vi "Parameter XML Write (ni-AIM).vi"(8 "error in":errorcluster, 10 "Parameter Array":T1[](array[typedef]), 11 "parameter file in":refnum<k24>) -> (0 "error out":errorcluster, 3 "parameter file out":refnum<k24>)   [LabVIEW 2020]
uses:
  Controls/Database_Array.ctl
  Controls/Encoding.ctl
  C:/Users/Administrator/Desktop/GIT/Ballard-Arinc-429-XML-Generator/Source/Assemblies/Aim_Parameter_ni/bin/Debug/AIM_429_Parameter_ni.dll
  Assemblies/Aim_Parameter_ni/bin/Debug/AIM_429_Parameter_ni.dll
  Libraries/Aim_Parameter_ni/_tyedefs/label_type.ctl
  Libraries/Aim_Parameter_ni/_tyedefs/parameter_type.ctl
  <userlib>/_OpenG.lib/array/array.llb/Remove Duplicates from 1D Array (I32)__ogtk.vi
  <userlib>/_OpenG.lib/array/array.llb/Filter 1D Array with Scalar (I32)__ogtk.vi
  <userlib>/_OpenG.lib/array/array.llb/Index 1D Array Elements (Variant)__ogtk.vi
  Libraries/Aim_Parameter_ni/AIM_429_Parameter_ni.lvlib
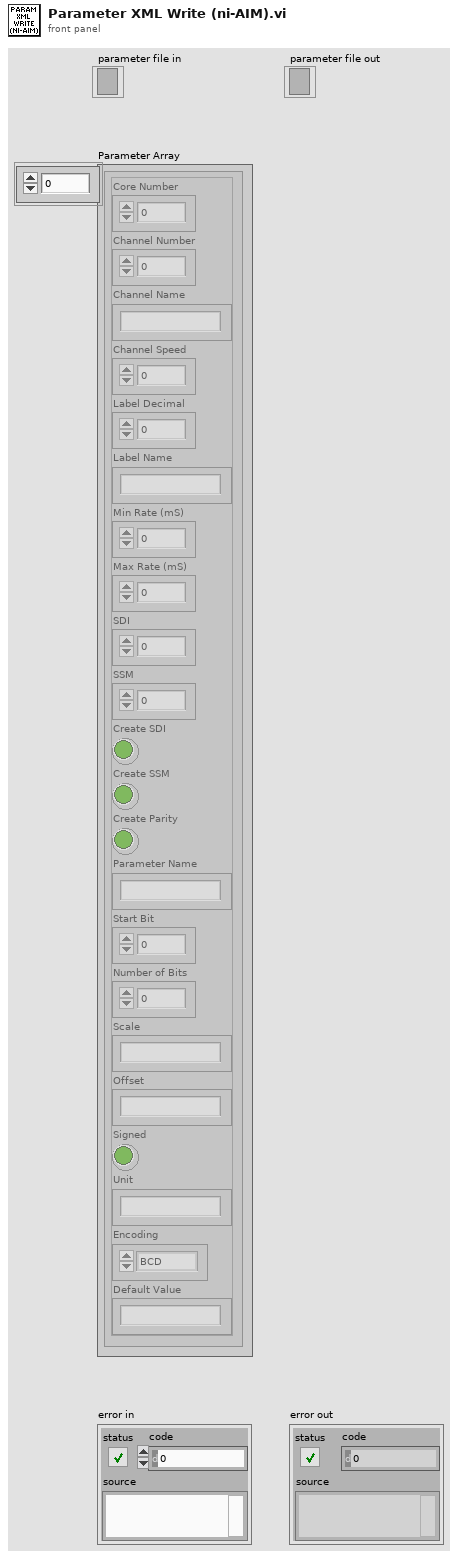
[diagram p1: front panel]
types:
  T1 = typedef "Database_Array.ctl" = cluster{"Core Number":i32, "Channel Number":i32, "Channel Name":string, "Channel Speed":i32, "Label Decimal":i32, "Label Name":string, "Min Rate (mS)":i32, "Max Rate (mS)":i32, "SDI":i32, "SSM":i32, "Create SDI":bool, "Create SSM":bool, "Create Parity":bool, "Parameter Name":string, "Start Bit":i32, "Number of Bits":i32, "Scale":string, "Offset":string, "Signed":bool, "Unit":string, "Encoding":T2, "Default Value":string}
  T2 = typedef "Encoding.ctl" = enum16{"BCD", "BNR", "Discrete"}
  T3 = typedef "AIM_429_Parameter_ni.lvlib/label_type.ctl" = cluster{"createParityChannel":bool, "createSDIChannel":bool, "createSSMChannel":bool, "createTimestampChannel":bool, "labelDecimal":i32, "labelDecimalSpecified":bool, "labelOctal":i32, "labelOctalSpecified":bool, "sdi":i32, "transferType":i32, "period":i32}
  T4 = typedef "AIM_429_Parameter_ni.lvlib/parameter_type.ctl" = cluster{"defaultValue":dbl, "encoding":i32, "name":string, "numberOfBits":i32, "offset":dbl, "scale":dbl, "signed":bool, "startBit":i32, "unit":string}
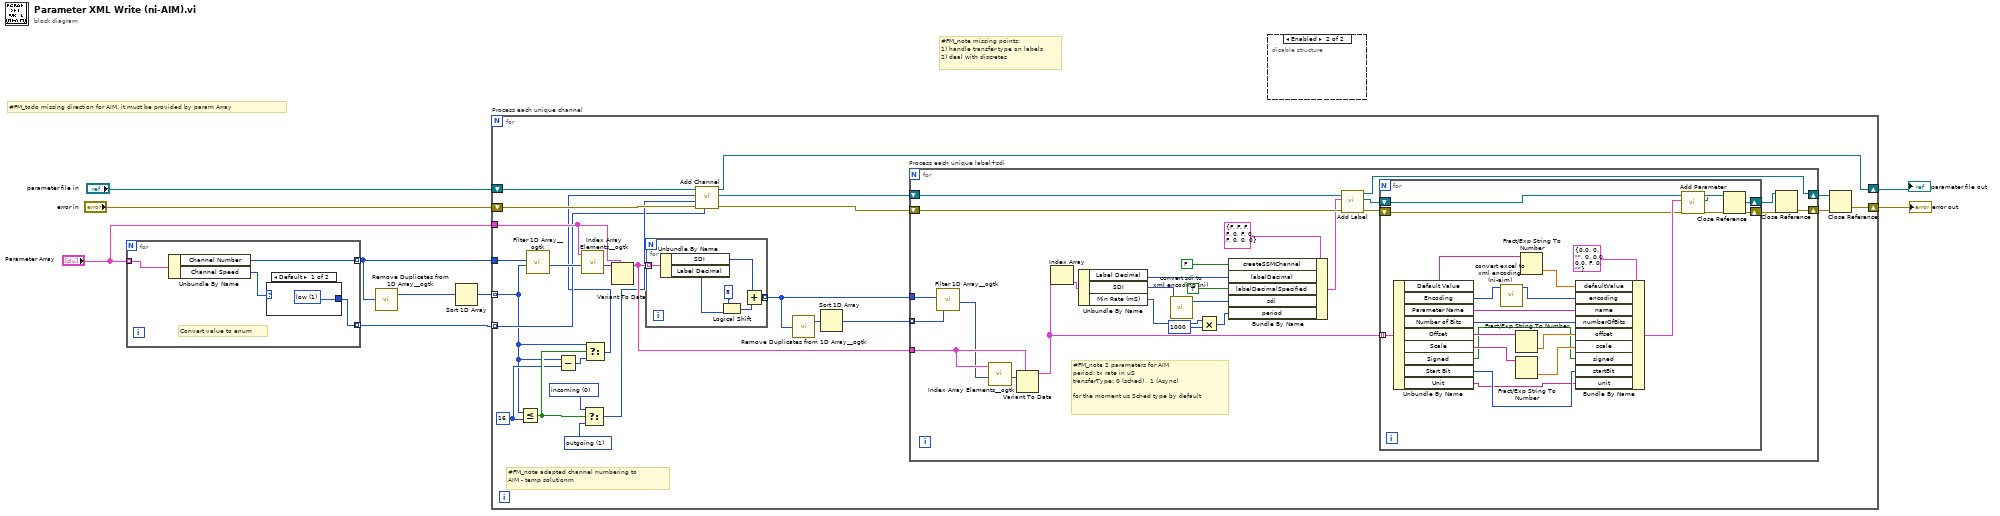
[diagram p0: block diagram]
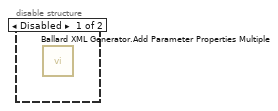
[diagram p2: hidden frame]
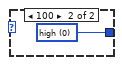
[diagram p3: hidden frame]
diagram:
  # "#FM_todo missing direction for AIM, it must be provided by param Array"
  # "#FM_note missing points:\n1) handle transfer type on labels\n2) deal with discretes"
  n1 = for {
    tunnel: [w13] -> w6 mode=indexing
    tunnel: "Parameter Array" -> [w12] mode=indexing
    tunnel: [w10] -> w1 mode=indexing
    # "Convert value to enum"
    n2 = Unbundle By Name(w12) -> ("Channel Number"=w13:i32, "Channel Speed"=w11:i32)
    n3 = case shown="Default" w11 {
      tunnel: [w14 w15] -> w10
      frame Default {
        w14 = 1 items=["high", "low"] ("speed (high)")
      }
      frame 100 {
        w15 = 0 items=["high", "low"] ("speed (high)")
      }
    }
  }
  n4 = call-poly <userlib>:"Remove Duplicates from 1D Array__ogtk.vi"("Input Array"=w6) -> ("Output Array"=w8:i32[])  [unwired: 1 out]
  n5 = Sort 1D Array(array=w8) -> (sorted array=w9:i32[])
  n6 = for "Process each unique channel" {
    tunnel: w9 -> [w17] mode=indexing
    tunnel: w6 -> [w40]
    tunnel: "Parameter Array" -> [w39]
    shift-right: [w37] -> w3
    shift-left: "parameter file in" -> [w38]
    shift-right: [w35] -> w2
    shift-left: "error in" -> [w36]
    tunnel: w1 -> [w21] mode=indexing
    w24 = 1 items=["incoming", "outgoing"] ("direction")
    w23 = 0 items=["incoming", "outgoing"] ("direction")
    w18 = 16 ("y")
    # "#FM_note adapted channel numbering to \nAIM - temp solutionm"
    n7 = Less Or Equal?(x=w17, y=w18) -> (x <= y?=w20:bool)
    n8 = call-poly <userlib>:"Filter 1D Array__ogtk.vi"("items to filter"=w17, "array"=w40) -> ("filtered item indices"=w31:i32[])  [unwired: 4 in, 1 out]
    n9 = Subtract(x=w17, y=w18) -> (x-y=w19:i32)
    n10 = call-poly <userlib>:"Index Array Elements__ogtk.vi"("indices"=w31, "array"=w39) -> ("elements"=w32:variant[])  [unwired: 9 in]
    n11 = Select(t=w23, s=w20, f=w24) -> (s? t:f=w22:i32)
    n12 = Select(t=w17, s=w20, f=w19) -> (s? t:f=w16:i32)
    n13 = Variant To Data(type=w39, Variant=w32) -> (data=w30:T1[])  [unwired: 1 in, 1 out]
    n14 = for {
      tunnel: w30 -> [w46] mode=indexing
      tunnel: [w42] -> w29 mode=indexing
      n15 = Unbundle By Name(w46) -> ("SDI"=w41:i32, "Label Decimal"=w43:i32)
      n16 = Logical Shift(y=i16 8, x=w43) -> (x << y=w45:i32)
      n17 = Add(x=w41, y=w45) -> (x+y=w42:i32)
    }
    n18 = call "Add Channel.vi"("speed (high)"=w21, "error in"=w36, "direction (incoming)"=w22, "hardwareChannel"=w16, "parameter file in"=w38) -> ("error out"=w27:errorcluster, "new channel"=w28:refnum<k24>, "parameter file out"=w37:refnum<k24>)  [unwired: 4 in]
    n19 = call-poly <userlib>:"Remove Duplicates from 1D Array__ogtk.vi"("Input Array"=w29) -> ("Output Array"=w34:i32[])  [unwired: 1 out]
    n20 = Sort 1D Array(array=w34) -> (sorted array=w33:i32[])
    n21 = for "Process each unique label+sdi" {
      tunnel: w33 -> [w70] mode=indexing
      tunnel: w29 -> [w71]
      tunnel: w30 -> [w68]
      shift-right: [w66] -> w25
      shift-left: w28 -> [w67]
      shift-right: [w53] -> w26
      shift-left: w27 -> [w65]
      # "#FM_note 2 parameters for AIM\nperiod: tx rate in uS\ntransferType: 0 (sched) , 1 (Async)\n\nfor the moment us Sched type by default"
      n22 = call-poly <userlib>:"Filter 1D Array__ogtk.vi"("items to filter"=w70, "array"=w71) -> ("filtered item indices"=w52:i32[])  [unwired: 4 in, 1 out]
      n23 = call-poly <userlib>:"Index Array Elements__ogtk.vi"("indices"=w52, "array"=w68) -> ("elements"=w69:variant[])  [unwired: 9 in]
      n24 = Variant To Data(type=w68, Variant=w69) -> (data=w56:T1[])  [unwired: 1 in, 1 out]
      n25 = Index Array(array=w56) -> (element=w62:T1)  [unwired: 1 in]
      n26 = Unbundle By Name(w62) -> ("Label Decimal"=w59:i32, "SDI"=w51:i32, "Min Rate (mS)"=w49:i32)
      n27 = call "convert sdi to xml encoding (ni).vi"("SDI"=w51) -> ("xml sdi format"=w50:i32)  [unwired: 10 in]
      n28 = Multiply(x=w49, y=1000) -> (x*y=w47:i32)
      n29 = Bundle By Name(cluster=T3 {"createParityChannel"=FALSE, "createSDIChannel"=FALSE, "createSSMChannel"=FALSE, "createTimestampChannel"=FALSE, "labelDecimal"=0, "labelDecimalSpecified"=FALSE, "labelOctal"=0, "labelOctalSpecified"=FALSE, "sdi"=0, "transferType"=0, "period"=0} ("label configuration"), "createSSMChannel"=FALSE, "labelDecimal"=w59, "labelDecimalSpecified"=TRUE, "sdi"=w50, "period"=w47) -> (w63:T3)
      n30 = call "Add Label.vi"("error in"=w65, "label configuration"=w63, "channel in"=w67) -> ("error out"=w58:errorcluster, "new label"=w57:refnum<k24>, "channel out"=w66:refnum<k24>)  [unwired: 6 in]
      n31 = for {
        shift-right: [w89] -> w55
        shift-left: w58 -> [w86]
        shift-right: [w92] -> w54
        shift-left: w57 -> [w93]
        tunnel: w56 -> [w74] mode=indexing
        n32 = Unbundle By Name(w74) -> ("Default Value"=w85:string, "Encoding"=w73:T2, "Parameter Name"=w78:string, "Number of Bits"=w79:i32, "Offset"=w83:string, "Scale"=w81:string, "Signed"=w77:bool, "Start Bit"=w76:i32, "Unit"=w75:string)
        n33 = call "convert excel to xml encoding (ni-aim).vi"("excel encoding"=w73) -> ("xml encoding"=w72:i32)  [unwired: 10 in]
        n34 = Fract/Exp String To Number(string=w83) -> (number=w82:dbl)  [unwired: 3 in, 1 out]
        n35 = Fract/Exp String To Number(string=w81) -> (number=w80:dbl)  [unwired: 3 in, 1 out]
        n36 = Fract/Exp String To Number(string=w85) -> (number=w84:dbl)  [unwired: 3 in, 1 out]
        n37 = Bundle By Name(cluster=T4 {"defaultValue"=0.0, "encoding"=0, "name"="", "numberOfBits"=0, "offset"=0.0, "scale"=0.0, "signed"=FALSE, "startBit"=0, "unit"=""} ("parameter configuration"), "defaultValue"=w84, "encoding"=w72, "name"=w78, "numberOfBits"=w79, "offset"=w82, "scale"=w80, "signed"=w77, "startBit"=w76, "unit"=w75) -> (w87:T4)
        n38 = call "Add Parameter.vi"("error in"=w86, "parameter configuration"=w87, "label in"=w93) -> ("error out"=w90:errorcluster, "new parameter"=w91:refnum<k24>, "label out"=w92:refnum<k24>)  [unwired: 6 in]
        n39 = Close Reference(reference=w91, error in (no error)=w90) -> (error out=w89:errorcluster)
      }
      n40 = Close Reference(reference=w54, error in (no error)=w55) -> (error out=w53:errorcluster)
    }
    n41 = Close Reference(reference=w25, error in (no error)=w26) -> (error out=w35:errorcluster)
  }
  "parameter file out" <- w3
  "error out" <- w2
  n42 = disable-structure shown="Enabled" {
    frame Disabled {
      n43 = call "Ballard XML Generator.Add Parameter Properties Multiple.vi"() -> ()  [unwired: 15 in, 1 out]
    }
    frame Enabled {
    }
  }
